vi "Find and Highlight Event Frames.vi"(8 "error in":errorcluster, 10 "Event Name":string, 11 "VI Reference":refnum<vi>) -> (0 "error out":errorcluster, 3 "Found?":bool)   [LabVIEW 2020, in "Panther Dashboard.lvlib"]
uses:
  Panther Dashboard.lvlib
  <vilib>/Utility/traverseref.llb/TRef TravTarget.ctl
  0da81d79-2fdf-41a2-a54a-73900cac0a2f.vi
  <vilib>/Utility/traverseref.llb/VI Scripting - Traverse.lvlib
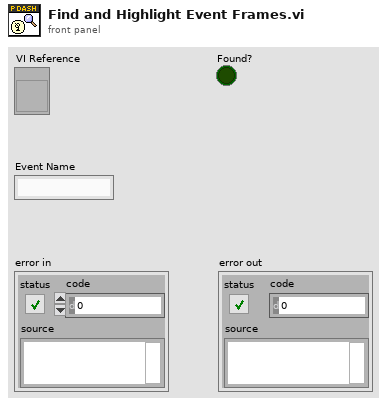
[diagram p1: front panel]
types:
  T1 = typedef "TRef TravTarget.ctl" = enum16{"FP", "BD", "Other"}
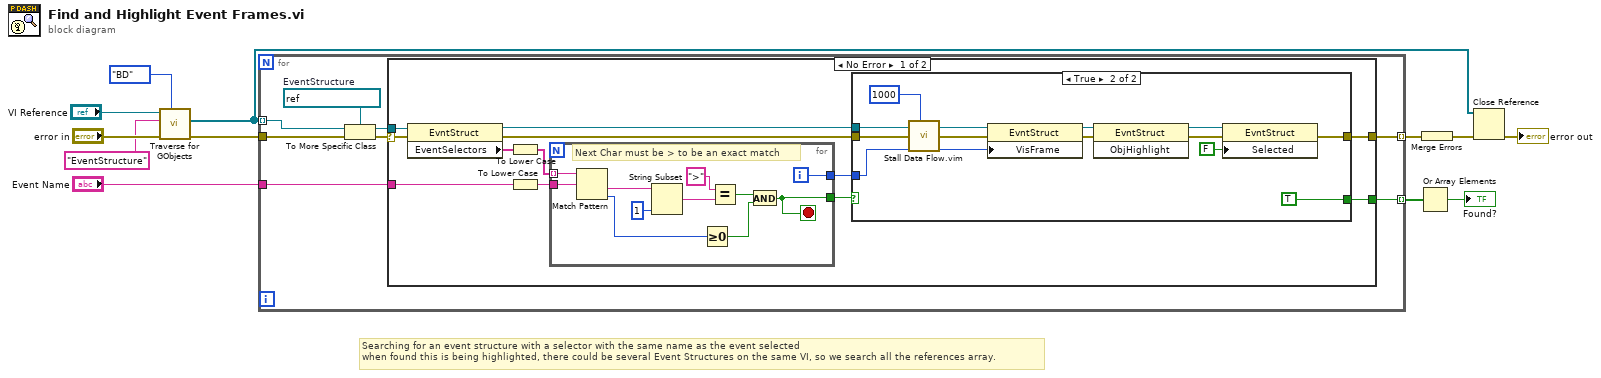
[diagram p0: block diagram]
diagram:
  # "Searching for an event structure with a selector with the same name as the event selected\nwhen found this is being highlighted, there could be several Event Structures on the same VI, so we search all the references array."
  n1 = call <vilib>:"Traverse for GObjects.vi"("Traverse Target"=TRef_TravTarget."BD", "error in (no error)"="error in", "Class Name"="EventStructure", "VI Refnum"="VI Reference") -> ("error out"=w10:errorcluster, "References"=w3:refnum<vi>[])  [unwired: 4 in, 2 out]
  n2 = for {
    tunnel: w3 -> [w17] mode=indexing
    tunnel: "Event Name" -> [w14]
    tunnel: w10 -> [w19]
    tunnel: [w18] -> w8 mode=indexing
    tunnel: [w13] -> w2 mode=indexing
    w16 = refnum<vi> refnum  # EventStructure
    n3 = To More Specific Class(target class=w16, reference=w17, error in=w19) -> (specific class reference=w15:refnum<vi>, error out=w20:errorcluster)
    n4 = case shown="No Error" w20 {
      selector: w20 -> [w32 _]
      tunnel: w15 -> [w27 _]
      tunnel: w14 -> [w28 _]
      tunnel: [w30 _] -> w18
      tunnel: [w21 _] -> w13
      frame No Error {
        n5 = property class="EvntStruct"(reference=w27, error in=w32) -> (reference out=w24:refnum<vi>, error out=w31:errorcluster, "EventSelectors"=w29:string[])
        n6 = To Lower Case(string=w29) -> (all lower case string=w23:string[])
        n7 = To Lower Case(string=w28) -> (all lower case string=w22:string)
        n8 = for {
          tunnel: w23 -> [w56] mode=indexing
          tunnel: w22 -> [w55]
          tunnel: [w54] -> w26
          tunnel: [w47] -> w25
          i -> [w54]
          stop <- w47 stop-if-true
          # "Next Char must be > to be an exact match"
          n9 = Match Pattern(string=w56, regular expression=w55) -> (after substring=w51:string, offset past match=w52:i32)  [unwired: 1 in, 2 out]
          n10 = String Subset(string=w51, length (rest)=1 ("length (rest)")) -> (substring=w50:string)  [unwired: 1 in]
          n11 = Greater Or Equal To 0?(x=w52) -> (x >= 0?=w53:bool)
          n12 = Equal?(x=">" ("y"), y=w50) -> (x = y?=w48:bool)
          n13 = And(x=w48, y=w53) -> (x .and. y?=w47:bool)
        }
        n14 = case shown="True" w25 {
          tunnel: w24 -> [_ w42]
          tunnel: w26 -> [_ w41]
          tunnel: w31 -> [w33 w36]
          tunnel: [w33 w43] -> w30
          tunnel: [_ TRUE ("Selected")] -> w21
          frame False {
          }
          frame True {
            n15 = call "Stall Data Flow.vim"("value in"=w36, "milliseconds to wait"=u32 1000) -> ("value out"=w35:errorcluster)  [unwired: 1 out]
            n16 = property class="EvntStruct"(reference=w42, error in=w35, "VisFrame"=w41) -> (reference out=w40:refnum<vi>, error out=w45:errorcluster)
            n17 = invoke class="EvntStruct" method="ObjHighlight"(reference=w40, error in=w45) -> (reference out=w39:refnum<vi>, error out=w44:errorcluster)  [unwired: 1 in, 1 out]
            n18 = property class="EvntStruct"(reference=w39, error in=w44, "Selected"=FALSE) -> (error out=w43:errorcluster)  [unwired: 1 out]
          }
        }
      }
      frame Error {
      }
    }
  }
  n19 = Or Array Elements(Boolean array=w2) -> (logical OR=→"Found?":bool)
  n20 = Merge Errors(w8) -> (w11:errorcluster)
  n21 = Close Reference(reference=w3, error in (no error)=w11) -> (error out=→"error out":errorcluster)
